vi "SerialWaitForStatusN.vi"(5 "error out 2":errorcluster, 7 "nStatusTries(400)":i32=400, 8 "VISA resource name(COM1)":refnum<visa-resource-name>="COM1") -> (0 "error out":errorcluster, 2 "Success":bool)   [LabVIEW 2010]
doc: "Sends STATUS command every 50 ms up to nStatusTries times.\nIf reply 'N' is received within nStatusTries times, then returns with Success = TRUE,\nelse returns with Success = FALSE."
uses:
  Instance           1 28Saved   SerialWaitForStatusN .vi
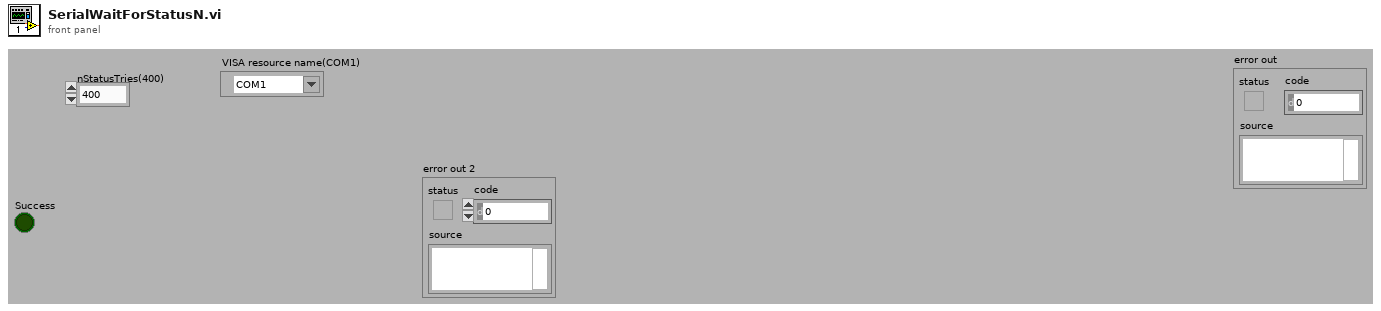
[diagram p1: front panel]
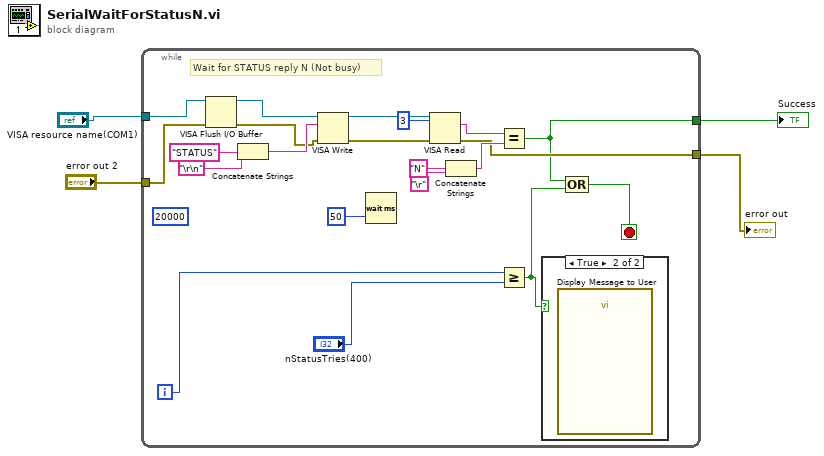
[diagram p0: block diagram]
diagram:
  n1 = while {
    tunnel: "VISA resource name(COM1)" -> [w12]
    tunnel: "error out 2" -> [w10]
    tunnel: [w14] -> w4
    tunnel: [w5] -> w1
    i -> [w6]
    stop <- w15 stop-if-true
    (unwired) 20000
    # "Wait for STATUS reply N (Not busy)"
    n2 = VISA Flush I/O Buffer(VISA resource name=w12, error in (no error)=w10) -> (VISA resource name out=w11:refnum<visa-resource-name>, error out=w9:errorcluster)  [unwired: 1 out]
    n3 = Concatenate Strings "Concatenate Strings"("STATUS" ("string"), "\r\n") -> (w23:string)
    n4 = VISA Write(VISA resource name=w11, write buffer=w23, error in (no error)=w9) -> (VISA resource name out=w22:refnum<visa-resource-name>, error out=w20:errorcluster)  [unwired: 1 out]
    n5 = Wait (ms)(milliseconds to wait=u32 50) -> ()  [unwired: 1 out]
    n6 = VISA Read(VISA resource name=w22, byte count=u32 3, error in (no error)=w20) -> (read buffer=w13:string, error out=w14:errorcluster)  [unwired: 2 out]
    n7 = Concatenate Strings("N" ("string"), "\r") -> (w19:string)
    n8 = Equal?(x=w13, y=w19) -> (x = y?=w5:bool)
    n9 = Greater Or Equal?(x=w6, y="nStatusTries(400)") -> (x >= y?=w7:bool)
    n10 = case shown="True" w7 {
      frame False {
      }
      frame True {
        n11 = call "Display Message to User"() -> ()  [unwired: 3 in, 9 out]
      }
    }
    n12 = Compound Arithmetic op=OR(w5, w7) -> (w15:bool)
  }
  "error out" <- w4
  "Success" <- w1
